vi "LVCAM Error.vi"(10 "error in":errorcluster, 11 "LVCAM Error in":refnum<class "LVCAM Error.lvclass">) -> (0 "error out":errorcluster)   [LabVIEW 2021, in "LVCAM.lvlib" / "LVCAM Error.lvclass"]
uses:
  LVCAM Error.lvclass
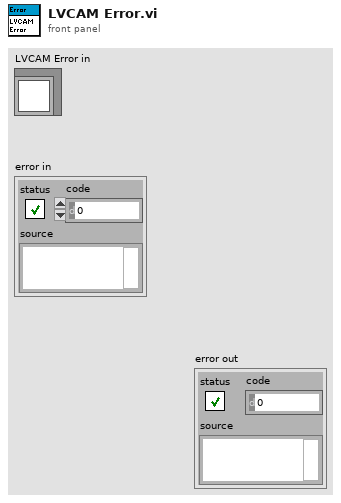
[diagram p1: front panel]
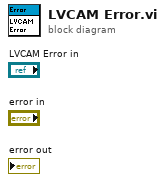
[diagram p0: block diagram]
diagram:
